vi "Parse Arguments.vi"(8 "error in (no error)":errorcluster, 11 "GPackCLI in":refnum<class "GPackCLI.lvclass">) -> (0 "error out":errorcluster, 3 "GPackCLI out":refnum<class "GPackCLI.lvclass">)   [LabVIEW 2020, in "GPackTools.lvlib" / "GPackCLI.lvclass"]
uses:
  GPackCLI.lvclass
  GPackCLI.lvclass/GPackCLI.ctl
  CLIAction/CLIAction.lvclass
  GPackTools.lvlib
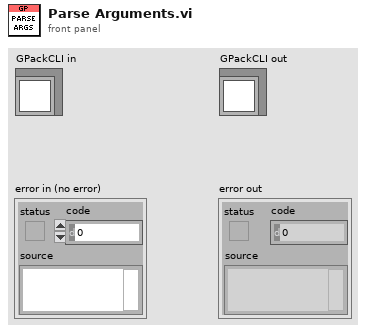
[diagram p1: front panel]
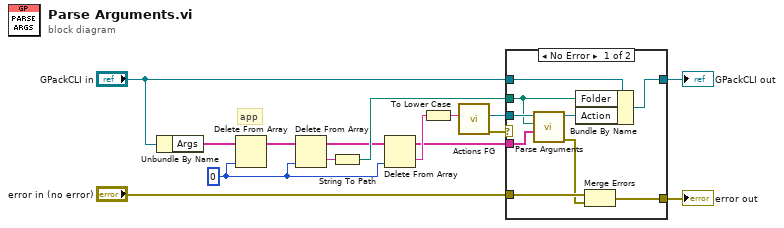
[diagram p0: block diagram]
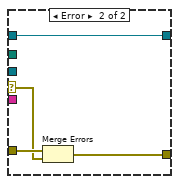
[diagram p2: hidden frame]
diagram:
  w10 = 0 ("index")
  # "app"
  n1 = Unbundle By Name("GPackCLI in") -> ("Args"=w8:string[])
  n2 = Delete From Array(array=w8, index=w10) -> (array with subset deleted=w11:string[])  [unwired: 1 in, 1 out]
  n3 = Delete From Array(array=w11, index=w10) -> (deleted portion=w15:string, array with subset deleted=w13:string[])  [unwired: 1 in]
  n4 = String To Path(string=w15) -> (path=w14:path)
  n5 = Delete From Array(array=w13, index=w10) -> (deleted portion=w12:string, array with subset deleted=w4:string[])  [unwired: 1 in]
  n6 = To Lower Case(string=w12) -> (all lower case string=w7:string)
  n7 = call "Actions FG.vi"("Action Name"=w7) -> ("error out"=w5:errorcluster, "Action"=w6:refnum<class "CLIAction.lvclass">)  [unwired: 9 in]
  n8 = case shown="No Error" w5 {
    selector: w5 -> [_ w26]
    tunnel: w14 -> [w21 _]
    tunnel: "GPackCLI in" -> [w24 w28]
    tunnel: w6 -> [w23 _]
    tunnel: w4 -> [w20 _]
    tunnel: "error in (no error)" -> [w19 w27]
    tunnel: [w17 w28] -> w2
    tunnel: [w16 w25] -> w1
    frame No Error {
      n9 = call-dynamic "Parse Arguments.vi"("Args"=w20, "Folder"=w21, "CLIAction in"=w23) -> ("error out"=w18:errorcluster, "CLIAction out"=w22:refnum<class "CLIAction.lvclass">)  [unwired: 7 in]
      n10 = Bundle By Name(cluster=w24, "Folder"=w21, "Action"=w22) -> (w17:refnum<class "GPackCLI.lvclass">)
      n11 = Merge Errors(w19, w18) -> (w16:errorcluster)
    }
    frame Error {
      n12 = Merge Errors(w27, w26) -> (w25:errorcluster)
    }
  }
  "error out" <- w1
  "GPackCLI out" <- w2
